vi "Angle Calc_Individual Process R2.vi"(0 "Angle to Pixel Ratios":T3={"Horizontal Angle / Px Ratio"=0.09917687, "Vertical Angle / Px Ratio"=0.10003997}, 1 "Previous Angles":sgl[](array[numeric])=[93.87193, 100.424255, 106.972824], 5 "Num of Beacons":i8=5, 7 "Beacon Coordinates - Image":T2={"Beacon Position - X px"=[315.0, 370.0, 425.0], "Beacon Position - Y px"=[207.0, 206.0, 205.0]}, 9 "Current Servo Angle":dbl=90.0 format="%#_13g", 11 "Beacons Found (Bool Array)":bool[](array[boolean])=[TRUE, TRUE, TRUE], 12 "Previous Valid Angles":bool[](array[boolean])=[TRUE, TRUE, TRUE]) -> (3 "Servo Goal Angle":dbl, 4 "Valid Beacons (Bool Array)\nPosition Calc":bool[](array[boolean])=[TRUE, TRUE, TRUE], 6 "Num of Valid Beacons":i8=3, 8 "Angle Of Beacons \nRelative to Robot":sgl[](array[numeric])=[93.87193, 100.424255, 106.972824], 10 "Angles Valid\nServo Control":bool, 14 "Servo Tracking Debug":T1={"Servo Track Test\nAngles"=[93.87193, 100.424255, 106.972824], "Servo Goal Angle 2"=0.0, "Beacon Coordinates - Image 2"={"Beacon Position - X px"=[], "Beacon Position - Y px"=[]}}, 15 "Distance of Each\nBeacon from Line of Best Fit":sgl[](array[numeric])=[0.16650113, 0.33324653, 0.1666237])   [LabVIEW 2015]
uses:
  <vilib>/Analysis/NI_AALPro.lvlib
panel:
  in  "Max Previous\nAngle Dev.":sgl=16.0
  out "Beacon Coordinates\n - Image Centered":T2={"Beacon Position - X px"=[41.0, 107.0, 173.0], "Beacon Position - Y px"=[-51.0, -48.0, -46.0]}
  in  "Image Width":sgl=320.0 format="%#_13g"
  in  "Image Height":sgl=240.0 format="%#_13g"
  in  "Servo Middle\nAngleThreshold":dbl=4.0 format="%#_13g"
  out "Intercept":sgl=-52.386364 format="%#_13g"
  out "Angle Of Beacons \nRelative to Center (servo)":sgl[](array[numeric])=[3.8719318, 10.424257, 16.972828]
  out "Normalized Center of\nImage Angles":cluster{"X":sgl, "Y":sgl}={"X"=0.19651788, "Y"=-5.2332215} {"Y" format="%#_13g"; "X" format="%#_13g"}
  out "Beacon delta Angles":cluster{"X Angle":sgl[], "Y Angle":sgl[]}={"X Angle"=[4.0656266, 10.613175, 17.156971], "Y Angle"=[-5.0853934, -4.8352323, -4.585181]}
  out "Normalized Center of\nImage Coordinates":cluster{"X":sgl, "Y":sgl}={"X"=1.9814891, "Y"=-52.31131} {"Y" format="%#_13g"; "X" format="%#_13g"}
  out "Perpendicular Slope":sgl=-26.4 format="%#_13g"
  out "Normalized Beacon Coordinates":T4={"Beacon Position - X"=[-50.83362, -48.333008, -45.833496], "Beacon Position - Y"=[40.9937, 107.01261, 172.99368]}
  in  "DeviationThreshold":sgl=10.0 format="%#_13g"
  out "Slope":sgl=0.03787879 format="%#_13g"
  in  "Slope Threshold":sgl=10.0 format="%#_13g"
  # "CALIBRATION"
  # "INPUTS"
  # "INTERMEDIATE VARIABLE VALUES"
  # "FILTER THRESHOLDS"
  # "OUTPUT VALUES"
  # "IMPORTANT: This \nThreshold will be used\nto determine if center \nangle is within \n\"Tracking\" Range\n*update: currently not\nreally used.."
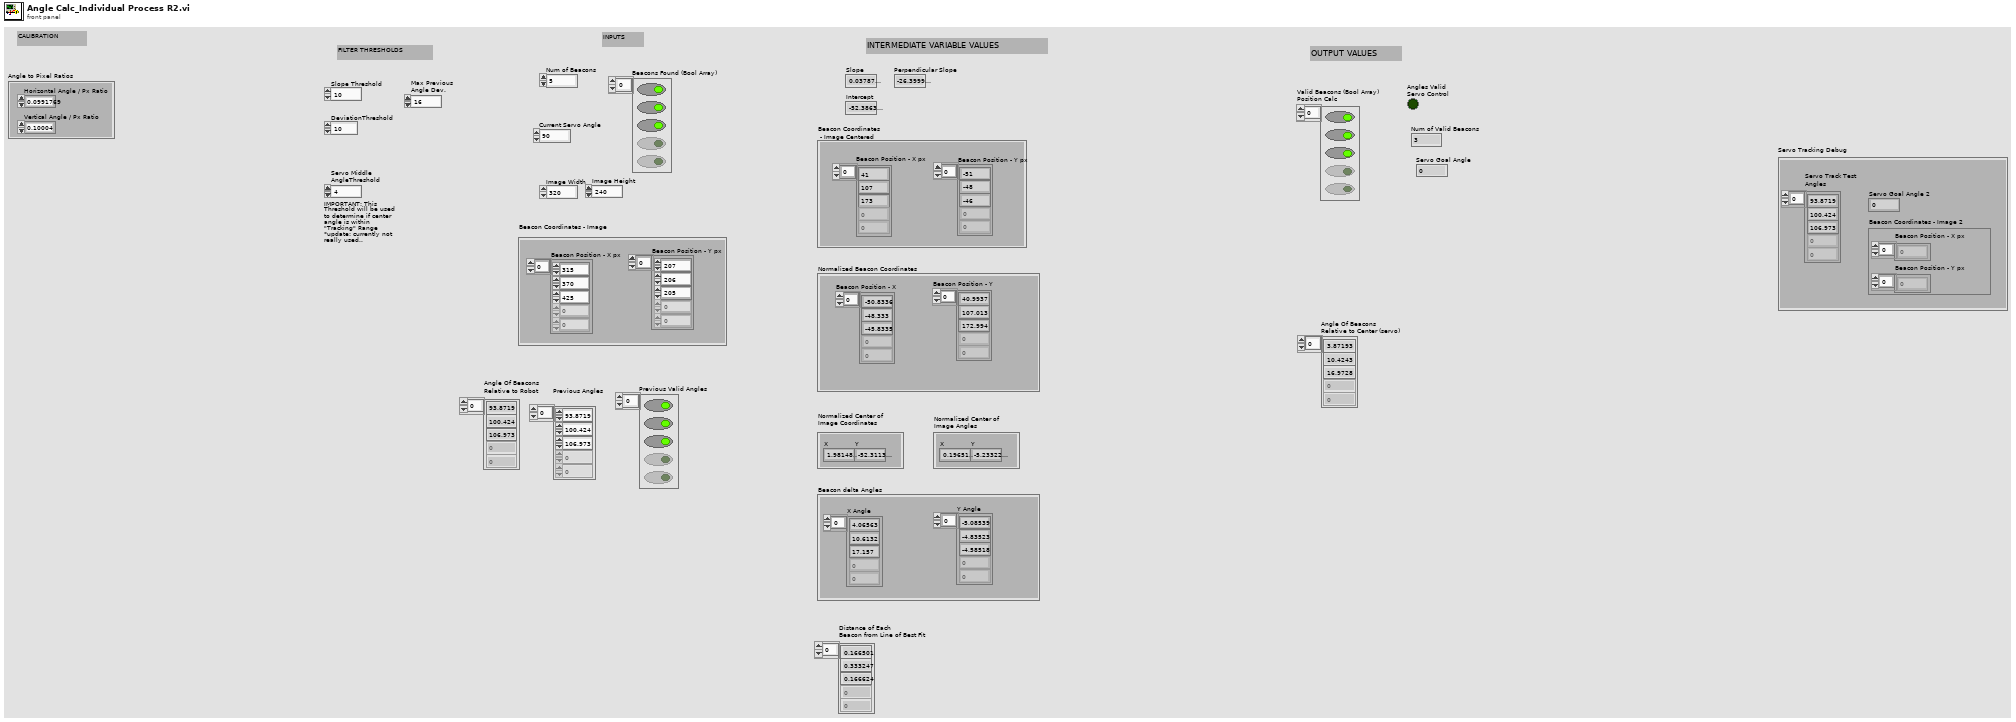
[diagram p1: front panel]
types:
  T1 = cluster{"Servo Track Test\nAngles":sgl[], "Servo Goal Angle 2":dbl, "Beacon Coordinates - Image 2":cluster{"Beacon Position - X px":sgl[], "Beacon Position - Y px":sgl[]}}
  T2 = cluster{"Beacon Position - X px":sgl[], "Beacon Position - Y px":sgl[]}
  T3 = cluster{"Horizontal Angle / Px Ratio":sgl, "Vertical Angle / Px Ratio":sgl}
  T4 = cluster{"Beacon Position - X":sgl[], "Beacon Position - Y":sgl[]}
  T5 = cluster{dbl[], "Current Servo Angle":dbl, "Beacon Coordinates - Image":cluster{"Beacon Position - X px":sgl[], "Beacon Position - Y px":sgl[]}}
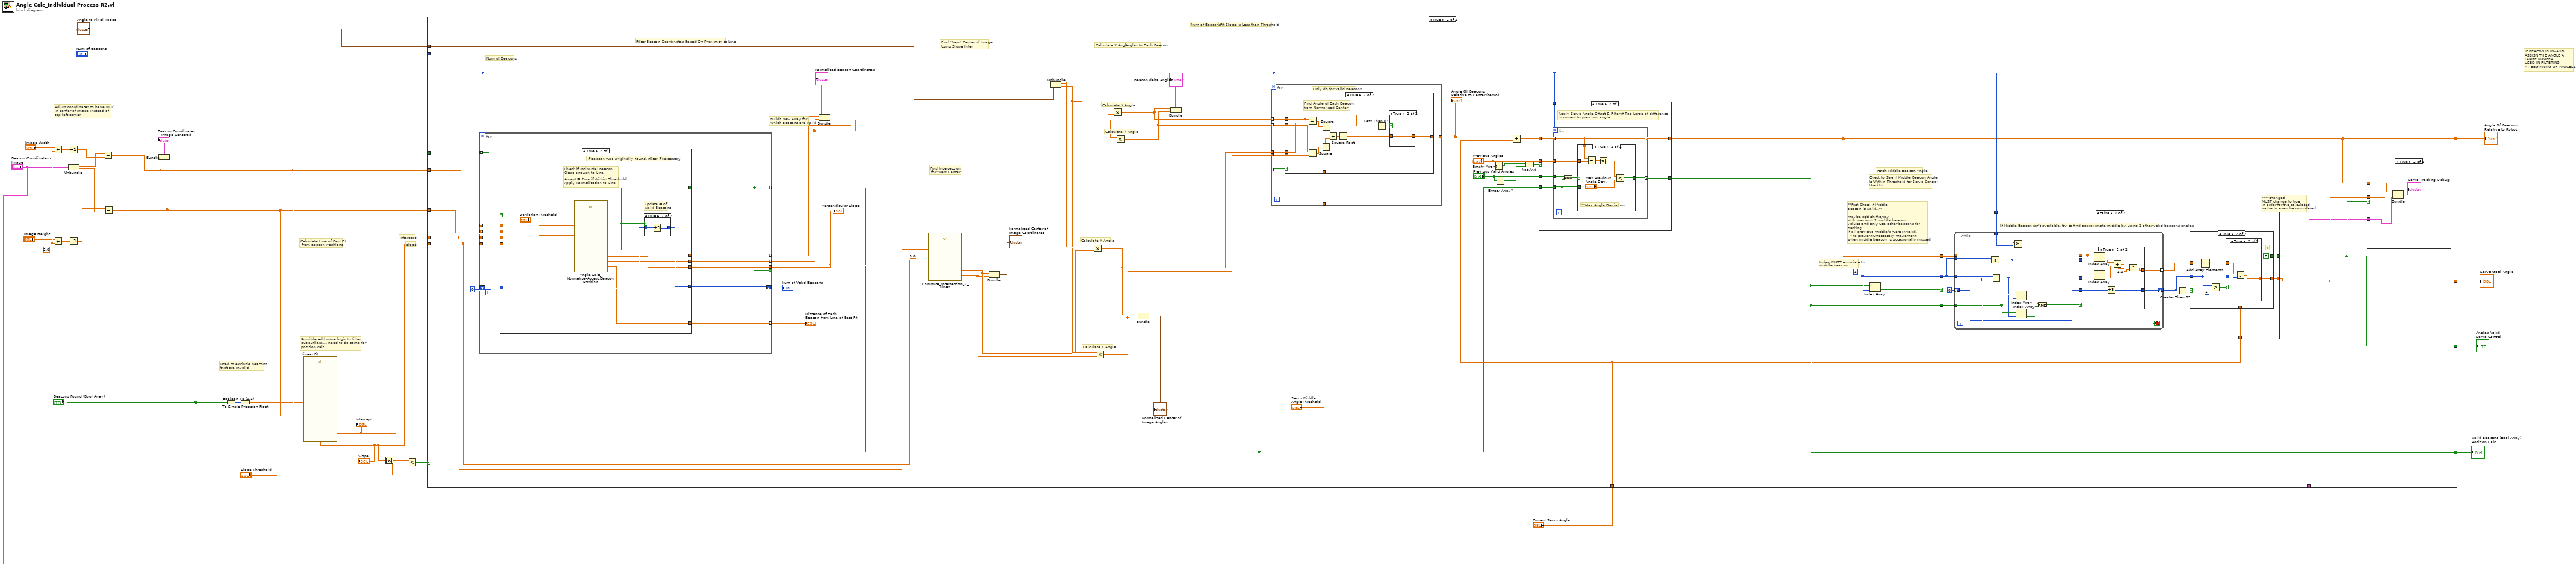
[diagram p0: block diagram]
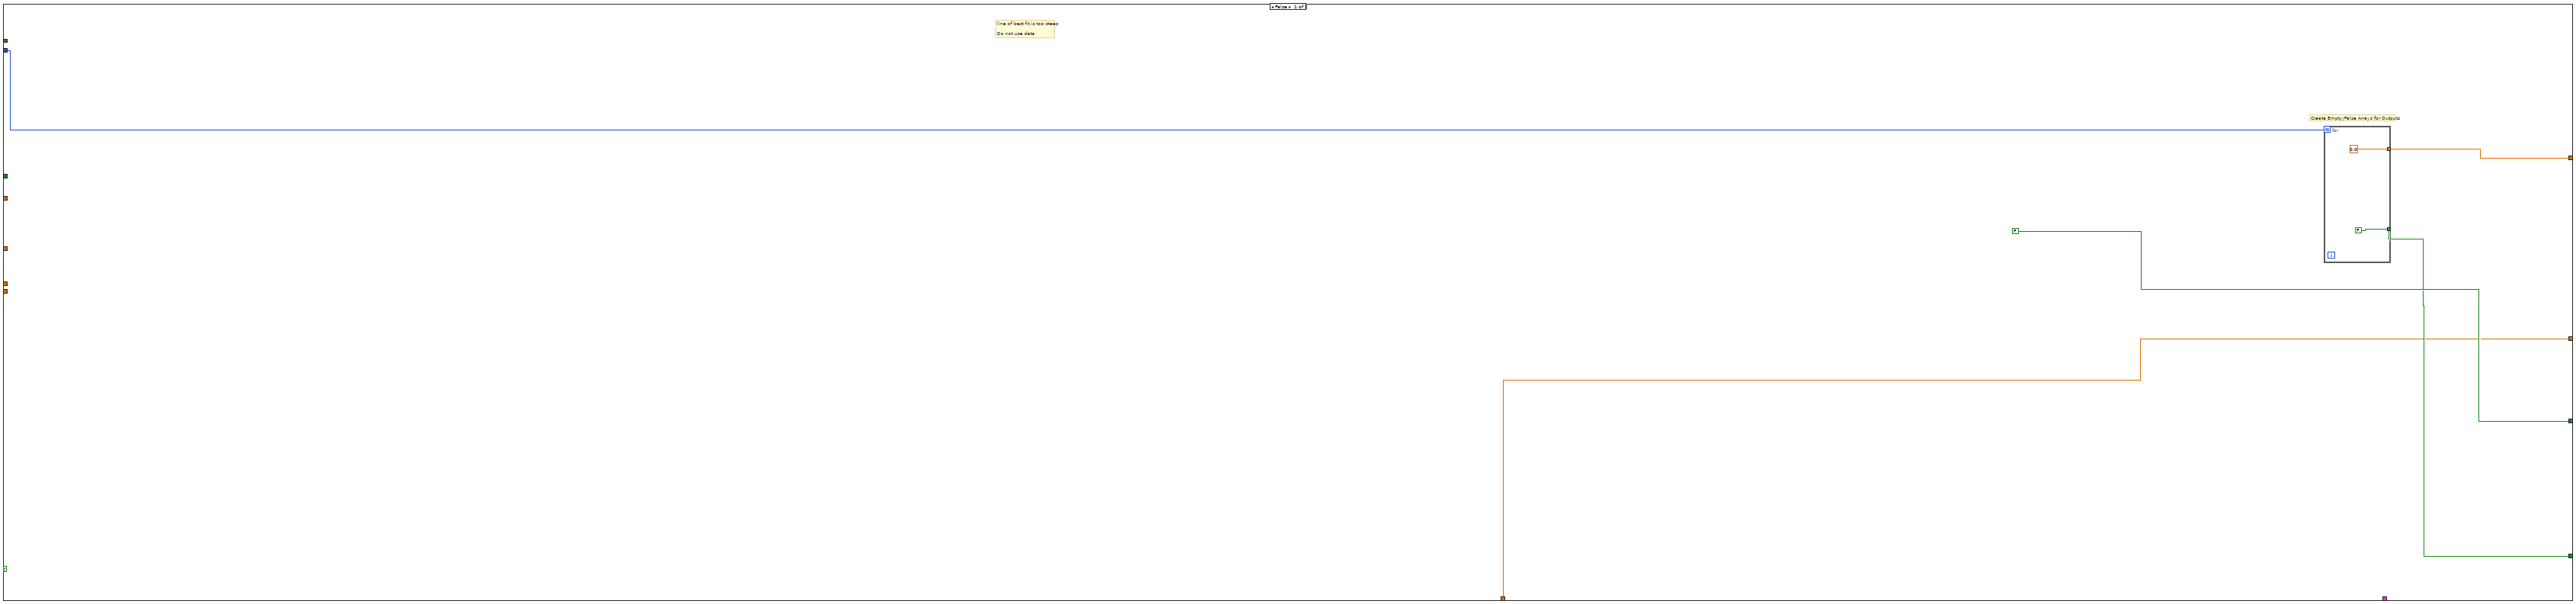
[diagram p2: hidden frame]
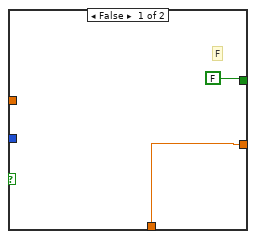
[diagram p6: hidden frame]
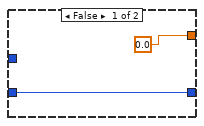
[diagram p8: hidden frame]
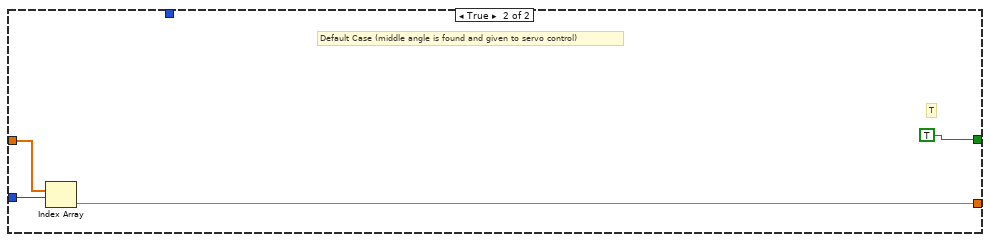
[diagram p9: hidden frame]
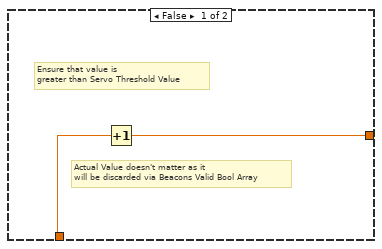
[diagram p10: hidden frame]
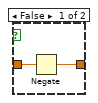
[diagram p11: hidden frame]
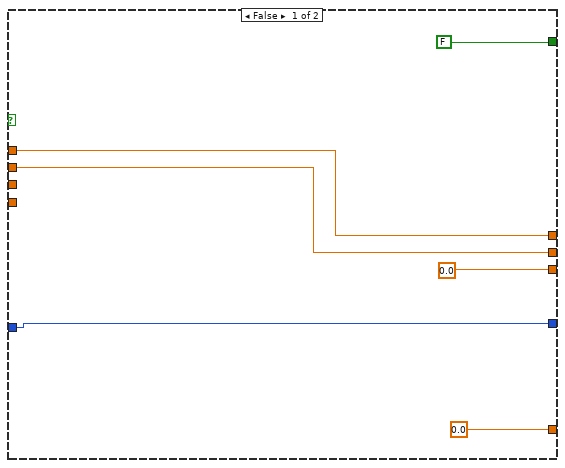
[diagram p12: hidden frame]
diagram:
  w14 = sgl 2.0
  # "Possible add more logic to filter\nout outliers.... need to do same for\nposition calc"
  # "IF BEACON IS INVALID\nASSISN THE ANGLE A\nLARGE NUMBER\nUSED IN FILTERING \nAT BEGINNING OF PROCESS"
  # "Adjust coordinates to have (0,0) \nin center of image instead of \ntop left corner"
  # "Calculate Line of Best Fit\n from Beacon Positions"
  # "slope"
  # "intercept"
  # "Used to exclude beacons \nthat are invalid"
  n1 = Divide(x="Image Width", y=w14) -> (x/y=w16:sgl)
  n2 = Divide(x="Image Height", y=w14) -> (x/y=w15:sgl)
  n3 = Decrement(x=w16) -> (x-1=w12:sgl)
  n4 = Decrement(x=w15) -> (x-1=w11:sgl)
  n5 = Unbundle("Beacon Coordinates - Image") -> ("Beacon Position - X px"=w19:sgl[], "Beacon Position - Y px"=w18:sgl[])
  n6 = Subtract(x=w19, y=w12) -> (x-y=w7:sgl[])
  n7 = Subtract(x=w11, y=w18) -> (x-y=w6:sgl[])
  n8 = Bundle(w7, w6) -> (→"Beacon Coordinates\n - Image Centered":cluster{sgl[], sgl[]})  [unwired: 1 in]
  n9 = Boolean To (0,1)(Boolean="Beacons Found (Bool Array)") -> (0, 1=w24:i16[])
  n10 = To Single Precision Float(number=w24) -> (single precision float=w4:sgl[])
  n11 = call <vilib>:"Linear Fit.vi"("Y"=w6, "X"=w7, "Weight"=w4) -> ("slope"=w21:dbl, "intercept"=w22:dbl)  [unwired: 8 in, 3 out]
  "Slope" <- w21
  "Intercept" <- w22
  n12 = Absolute Value(x=w21) -> (abs(x)=w20:dbl)
  n13 = Less?(x=w20, y="Slope Threshold") -> (x < y?=w23:bool)
  n14 = case shown="True" w23 {
    tunnel: w21 -> [_ w76]
    tunnel: w22 -> [_ w75]
    tunnel: w7 -> [_ w78]
    tunnel: w6 -> [_ w77]
    tunnel: "Angle to Pixel Ratios" -> [_ w74]
    tunnel: "Num of Beacons" -> [w32 w60]
    tunnel: [w30 w49] -> w28
    tunnel: [FALSE w50] -> w27
    tunnel: [w31 w59] -> w26
    tunnel: "Beacons Found (Bool Array)" -> [_ w63]
    tunnel: [w29 w48] -> w3
    tunnel: "Current Servo Angle" -> [w29 w39]
    tunnel: "Beacon Coordinates - Image" -> [_ w47]
    frame False {
      # "Create Empty/False Arrays for Outputs"
      # "line of best fit is too steep\n\nDo not use data"
      n15 = for {
        N: w32 -> [_]
        tunnel: [FALSE] -> w31 mode=indexing
        tunnel: [sgl 0.0] -> w30 mode=indexing
      }
    }
    frame True {
      w61 = 2
      # "****changed\nMUST change to true\nin order for the calculated\nvalue to even be considered"
      # "**First Check if Middle\nBeacon is Valid..**\n\nmaybe add shift array\nwith previous 3 middle beacon\nvalues and only use other beacons for tracking\nif all previous middle's were invalid.\n-> to prevent unessesary movement\nwhen middle beacon is occasionally missed"
      # "Calculate X Angle"
      # "Index MUST associate to\nmiddle beacon"
      # "Fetch Middle Beacon Angle"
      # "Check to See if Middle Beacon Angle\nIs Within Threshold for Servo Control\nUsed to"
      # "Num of Beacons"
      # "Find dX and dY Angles to Each Beacon"
      # "Calculate Y Angle"
      # "Calculate X Angle"
      # "Calculate Y Angle"
      # "Calculate X Angle"
      # "Find Intersection\n for \"New Center\""
      # "Find \"New\" Center of Image\nUsing Slope Inter"
      # "Num of Beacons"
      # "Builds New Array for\nWhich Beacons are Valid"
      # "Filter Beacon Coordinates Based On Proximity to Line"
      # "If Line of Bestst Fit Slope is Less than Threshold"
      n16 = for {
        N: w60 -> [_]
        shift-right: [w190] -> w67
        shift-left: 0 -> [w195]
        tunnel: w75 -> [w194]
        tunnel: w76 -> [w193]
        tunnel: w78 -> [w192] mode=indexing
        tunnel: w77 -> [w191] mode=indexing
        tunnel: [w184] -> w36 mode=indexing
        tunnel: [w189] -> w56 mode=indexing
        tunnel: [w188] -> w55 mode=indexing
        tunnel: [w187] -> w37 mode=indexing
        tunnel: w63 -> [w186] mode=indexing
        tunnel: [w185] -> w38 if=w184
        n17 = case shown="True" w186 {
          tunnel: w195 -> [w197 w207]
          tunnel: w194 -> [_ w212]
          tunnel: w193 -> [_ w211]
          tunnel: w192 -> [w199 w210]
          tunnel: w191 -> [w200 w209]
          tunnel: [FALSE w208] -> w184
          tunnel: [w197 w206] -> w190
          tunnel: [w199 w205] -> w189
          tunnel: [w200 w204] -> w188
          tunnel: [sgl 0.0 w203] -> w185
          tunnel: [sgl 0.0 w202] -> w187
          frame False {
          }
          frame True {
            # "Update # of \nValid Beacons"
            # "Check if Indivudal Beacon\nClose enough to Line\n\nAccept = True if Within Threshold\nApply Normalization to Line"
            # "If Beacon was Originally Found, Filter if Necessary"
            n18 = call "Angle Calc_Normalize-Accept Beacon Position.vi"("slope"=w211, "Xin"=w210, "Deviation Threshold"="DeviationThreshold", "intercept"=w212, "Yin"=w209) -> ("Accept Beacon"=w208:bool, "Xout"=w205:sgl, "Distance"=w202:sgl, "Perpendicular Slope"=w203:sgl, "Yout"=w204:sgl)  [unwired: 6 in]
            n19 = case shown="True" w208 {
              tunnel: [w214 w215] -> w206
              tunnel: w207 -> [w214 w216]
              frame False {
              }
              frame True {
                n20 = Increment(x=w216) -> (x+1=w215:i32)
              }
            }
          }
        }
      }
      "Num of Valid Beacons" <- w67
      "Distance of Each\nBeacon from Line of Best Fit" <- w37
      "Perpendicular Slope" <- w38
      n21 = Bundle(w56, w55) -> (→"Normalized Beacon Coordinates":cluster{sgl[], sgl[]})  [unwired: 1 in]
      n22 = call "Compute_Intersection_2_Lines.vi"("m'"=w38, "b'"=0.0, "b"=w75, "m"=w76) -> ("Yint"=w57:sgl, "Xint"=w58:sgl)  [unwired: 6 in]
      n23 = Bundle("Xint"=w58, "Yint"=w57) -> (→"Normalized Center of\nImage Coordinates":cluster{"Xint":sgl, "Yint":sgl})  [unwired: 1 in]
      n24 = Unbundle(w74) -> ("Horizontal Angle / Px Ratio"=w65:sgl, "Vertical Angle / Px Ratio"=w64:sgl)
      n25 = Multiply(x=w65, y=w58) -> (x*y=w51:sgl)
      n26 = Multiply(x=w64, y=w57) -> (x*y=w52:sgl)
      n27 = Multiply(x=w65, y=w56) -> (x*y=w53:sgl[])
      n28 = Multiply(x=w55, y=w64) -> (x*y=w54:sgl[])
      n29 = Bundle(w51, w52) -> (→"Normalized Center of\nImage Angles":cluster{sgl, sgl})  [unwired: 1 in]
      n30 = Bundle(w53, w54) -> (→"Beacon delta Angles":cluster{sgl[], sgl[]})  [unwired: 1 in]
      n31 = for {
        N: w60 -> [_]
        tunnel: w53 -> [w166] mode=indexing
        tunnel: w54 -> [w165] mode=indexing
        tunnel: w51 -> [w164]
        tunnel: w52 -> [w163]
        tunnel: [w162] -> w40 mode=indexing
        tunnel: w36 -> [w161] mode=indexing
        tunnel: "Servo Middle\nAngleThreshold" -> [w160]
        # "Only do for Valid Beacons"
        n32 = case shown="True" w161 {
          tunnel: w166 -> [_ w171]
          tunnel: w165 -> [_ w175]
          tunnel: w164 -> [_ w174]
          tunnel: w163 -> [_ w173]
          tunnel: [w168 w169] -> w162
          tunnel: w160 -> [w167 _]
          frame False {
            # "Actual Value doesn't matter as it\nwill be discarded via Beacons Valid Bool Array"
            # "Ensure that value is \ngreater than Servo Threshold Value"
            n33 = Increment(x=w167) -> (x+1=w168:dbl)
          }
          frame True {
            # "Find Angle of Each Beacon \nfrom Normalized Center"
            n34 = Subtract(x=w171, y=w174) -> (x-y=w177:sgl)
            n35 = Subtract(x=w175, y=w173) -> (x-y=w176:sgl)
            n36 = Square(x=w176) -> (x^2=w179:sgl)
            n37 = Square(x=w177) -> (x^2=w180:sgl)
            n38 = Add(x=w180, y=w179) -> (x+y=w178:sgl)
            n39 = Square Root(x=w178) -> (sqrt(x)=w170:sgl)
            n40 = Less Than 0?(x=w171) -> (x < 0?=w172:bool)
            n41 = case shown="True" w172 {
              tunnel: w170 -> [w181 w183]
              tunnel: [w182 w183] -> w169
              frame False {
                n42 = Negate(x=w181) -> (-x=w182:sgl)
              }
              frame True {
              }
            }
          }
        }
      }
      "Angle Of Beacons \nRelative to Center (servo)" <- w40
      n43 = Empty Array?(array="Previous Angles") -> (empty?=w43:bool)
      n44 = Empty Array?(array="Previous Valid Angles") -> (empty?=w42:bool)
      n45 = Add(x=w40, y=w39) -> (x+y=w41:dbl[])
      n46 = Not And(1:w42, 2:w43) -> (0:w44:bool)
      n47 = case shown="True" w44 {
        tunnel: w60 -> [_ w87]
        tunnel: "Previous Angles" -> [_ w86]
        tunnel: "Previous Valid Angles" -> [_ w85]
        tunnel: w36 -> [w80 w84]
        tunnel: [w80 w83] -> w59
        tunnel: [w79 w82] -> w49
        tunnel: w41 -> [w79 w81]
        frame False {
        }
        frame True {
          # "Apply Servo Angle Offset & Filter if Too Large of difference\nin current to previous angle"
          n48 = for {
            N: w87 -> [_]
            tunnel: [w88] -> w82 mode=indexing
            tunnel: w86 -> [w93] mode=indexing
            tunnel: w85 -> [w90] mode=indexing
            tunnel: [w92] -> w83 mode=indexing
            tunnel: w84 -> [w89] mode=indexing
            tunnel: w81 -> [w88] mode=indexing
            n49 = And(x=w90, y=w89) -> (x .and. y?=w91:bool)
            n50 = case shown="True" w91 {
              tunnel: w93 -> [_ w100]
              tunnel: [w94 w96] -> w92
              tunnel: w88 -> [_ w97]
              tunnel: w89 -> [w94 _]
              frame False {
              }
              frame True {
                # "**Max Angle Deviation"
                n51 = Subtract(x=w97, y=w100) -> (x-y=w99:dbl)
                n52 = Absolute Value(x=w99) -> (abs(x)=w98:dbl)
                n53 = Less?(x=w98, y="Max Previous\nAngle Dev.") -> (x < y?=w96:bool)
              }
            }
          }
        }
      }
      n54 = Index Array(array=w59, index=w61) -> (element=w62:bool)
      n55 = case shown="False" w62 {
        tunnel: w61 -> [w114 w159]
        tunnel: w49 -> [w115 w158]
        tunnel: [w107 w157] -> w48
        tunnel: w59 -> [w113 _]
        tunnel: w60 -> [w111 _]
        tunnel: w39 -> [w106 _]
        tunnel: [w105 TRUE] -> w50
        frame False {
          # "If Middle Beacon isn't available, try to find approximate middle by using 2 other valid beacons angles"
          n56 = while {
            tunnel: w115 -> [w143]
            tunnel: w114 -> [w142]
            tunnel: w114 -> [w141]
            tunnel: w113 -> [w139]
            tunnel: [w134] -> w108 mode=indexing
            shift-right: [w133] -> w109
            shift-left: 0 -> [w132]
            tunnel: w111 -> [w129]
            i -> [w140]
            stop <- w131 stop-if-true
            n57 = Add(x=w142, y=w140) -> (x+y=w130:i32)
            n58 = Subtract(x=w141, y=w140) -> (x-y=w138:i32)
            n59 = Greater Or Equal?(x=w130, y=w129) -> (x >= y?=w131:bool)
            n60 = Index Array(array=w139, index=w130) -> (element=w137:bool)
            n61 = Index Array(array=w139, index=w138) -> (element=w136:bool)
            n62 = And(x=w137, y=w136) -> (x .and. y?=w135:bool)
            n63 = case shown="True" w135 {
              tunnel: w143 -> [_ w153]
              tunnel: w130 -> [_ w155]
              tunnel: w138 -> [_ w154]
              tunnel: [sgl 0.0 w149] -> w134
              tunnel: [w144 w147] -> w133
              tunnel: w132 -> [w144 w146]
              frame False {
              }
              frame True {
                n64 = Index Array(array=w153, index=w155) -> (element=w152:dbl)
                n65 = Index Array(array=w153, index=w154) -> (element=w151:dbl)
                n66 = Increment(x=w146) -> (x+1=w147:i32)
                n67 = Add(x=w152, y=w151) -> (x+y=w150:dbl)
                n68 = Divide(x=w150, y=sgl 2.0) -> (x/y=w149:dbl)
              }
            }
          }
          n69 = Greater Than 0?(x=w109) -> (x > 0?=w110:bool)
          n70 = case shown="True" w110 {
            tunnel: w109 -> [_ w122]
            tunnel: w108 -> [_ w121]
            tunnel: [w117 w119] -> w107
            tunnel: w106 -> [w117 _]
            tunnel: [FALSE FALSE] -> w105
            frame False {
              # "F"
            }
            frame True {
              # "T"
              n71 = Add Array Elements(numeric array=w121) -> (sum=w120:dbl)
              n72 = Greater?(x=w122, y=1) -> (0:w124:bool)
              n73 = case shown="True" w124 {
                tunnel: w122 -> [_ w128]
                tunnel: w120 -> [w125 w127]
                tunnel: [w125 w126] -> w119
                frame False {
                }
                frame True {
                  n74 = Divide(x=w127, y=w128) -> (x/y=w126:dbl)
                }
              }
            }
          }
        }
        frame True {
          # "Default Case (middle angle is found and given to servo control)"
          # "T"
          n75 = Index Array(array=w158, index=w159) -> (element=w157:dbl)
        }
      }
      n76 = case shown="True" w50 {
        tunnel: w49 -> [_ w104]
        tunnel: w48 -> [_ w103]
        tunnel: w47 -> [_ w102]
        frame False {
        }
        frame True {
          n77 = Bundle(w104, "Current Servo Angle"=w103, "Beacon Coordinates - Image"=w102) -> (→"Servo Tracking Debug":T5)  [unwired: 1 in]
        }
      }
    }
  }
  "Angle Of Beacons \nRelative to Robot" <- w28
  "Angles Valid\nServo Control" <- w27
  "Valid Beacons (Bool Array)\nPosition Calc" <- w26
  "Servo Goal Angle" <- w3
